vi "channel_producer.vi"   [LabVIEW 2020]
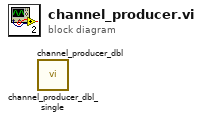
[diagram p0: block diagram]
diagram:
  n1 = call "channel_producer_dbl_single.vi"() -> ()  [unwired: 7 in, 2 out]
  n2 = call "channel_producer_dbl.vi"() -> ()  [unwired: 7 in, 2 out]
